vi "Get Download Progress.vi"(7 "Download Timeout (S)":u32, 8 "Error In":errorcluster, 11 "Download":T1) -> (0 "Error Out":errorcluster, 1 "Complete?":bool, 2 "Percent Complete":i32, 3 "Download":T1, 4 "Timeout?":bool)   [LabVIEW 2011, in "LVH-Toolbox.lvlib" / "LVH-Common.lvlib"]
doc: "Get progress of current download. If the download fails to progress during the timeout duration the download will be aborted.\n\nCall this VI in a loop after starting a download to monitor the download progress."
uses:
  LVH-Common.lvlib
  Private/Web/Type Defs/Download Task.ctl
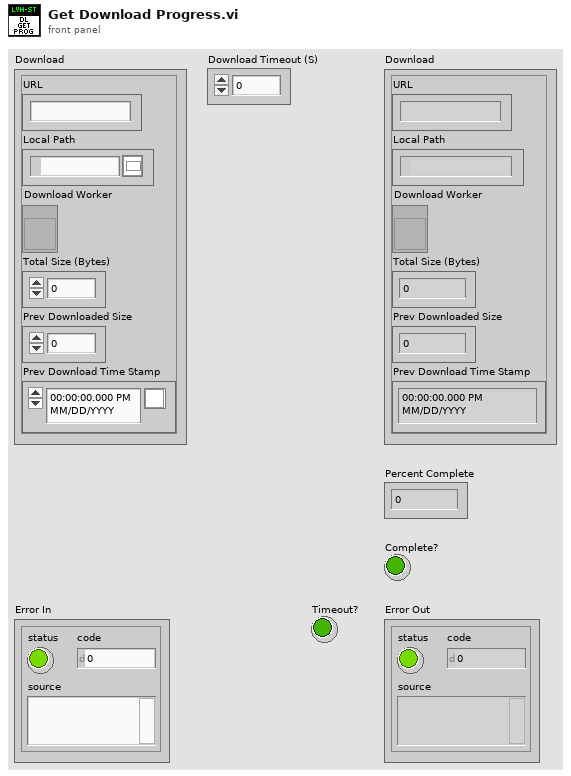
[diagram p1: front panel]
types:
  T1 = typedef "LVH-Toolbox.lvlib/LVH-Common.lvlib/Download Task.ctl" = cluster{"URL":string, "Local Path":path, "Download Worker":refnum<vi>, "Total Size (Bytes)":u64, "Prev Downloaded Size":u64, "Prev Download Time Stamp":timestamp}
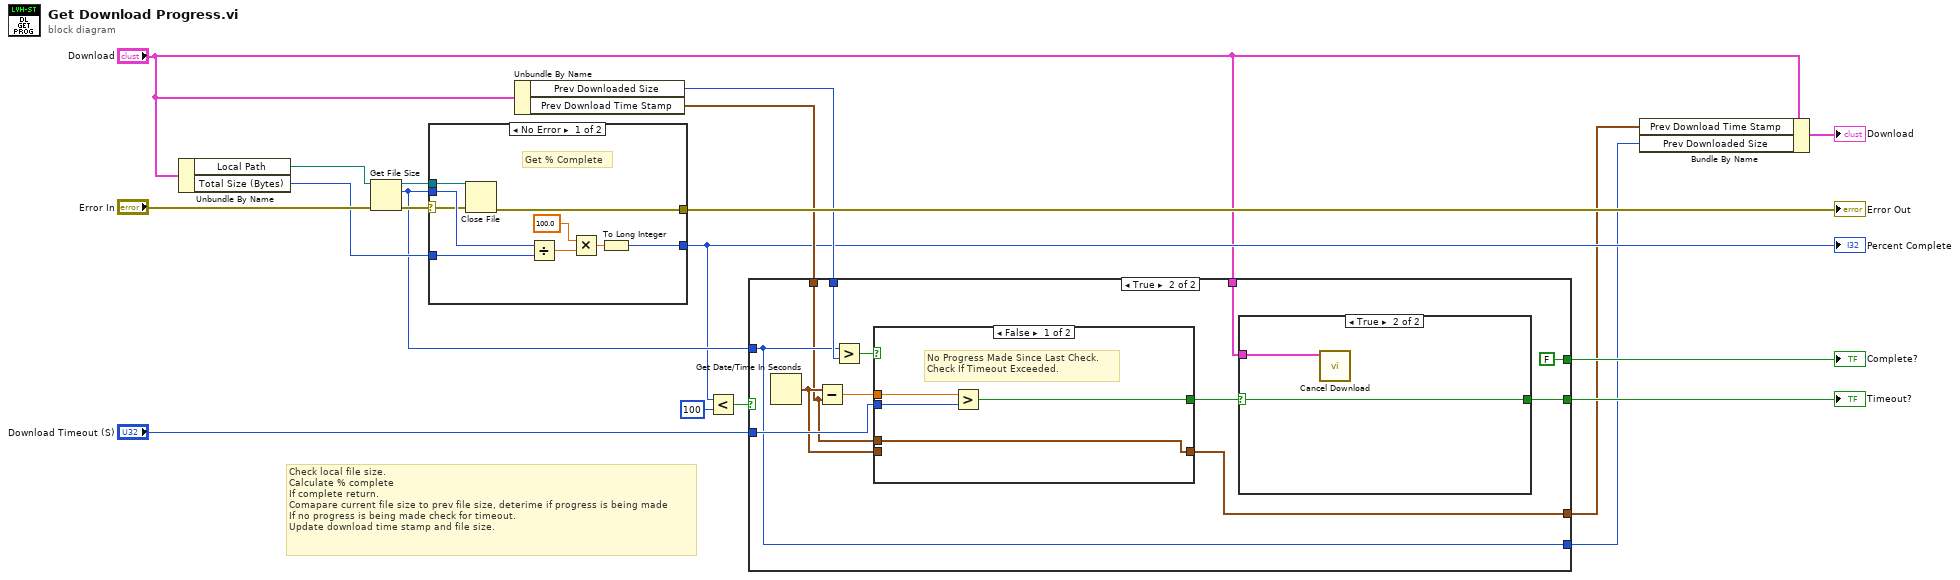
[diagram p0: block diagram]
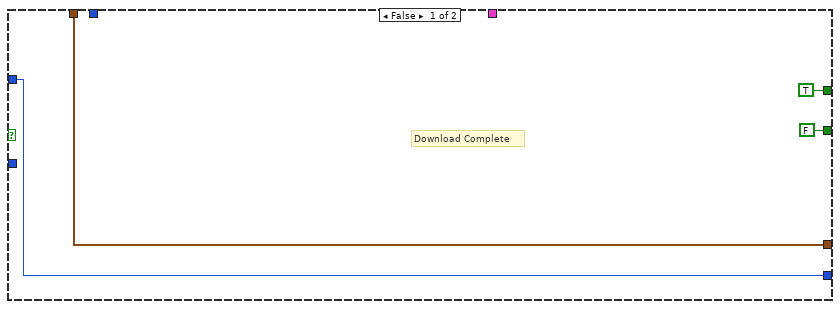
[diagram p2: hidden frame]
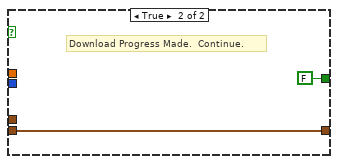
[diagram p4: hidden frame]
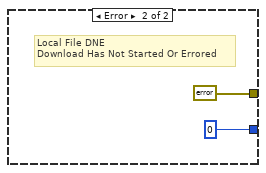
[diagram p5: hidden frame]
diagram:
  # "Check local file size.\nCalculate % complete\nIf complete return.\nComapare current file size to prev file size, deterime if progress is being made\nIf no progress is being made check for timeout.\nUpdate download time stamp and file size."
  n1 = Unbundle By Name("Download") -> ("Local Path"=w16:path, "Total Size (Bytes)"=w15:u64)
  n2 = Get File Size(file=w16, error in="Error In") -> (refnum out=w5:refnum<file>, size (in bytes)=w14:i64, 0:w17:errorcluster)
  n3 = case shown="No Error" w17 {
    selector: w17 -> [w21 _]
    tunnel: w14 -> [w28 _]
    tunnel: w5 -> [w24 _]
    tunnel: [w23 0] -> w8
    tunnel: [w22 errorcluster {"status"=FALSE, "code"=0, "source"=""} ("error out")] -> w18
    tunnel: w15 -> [w20 _]
    frame No Error {
      # "Get % Complete"
      n4 = Close File(refnum=w24, error in=w21) -> (error out=w22:errorcluster)  [unwired: 1 out]
      n5 = Divide(x=w28, y=w20) -> (x/y=w27:dbl)
      n6 = Multiply(x=100.0, y=w27) -> (x*y=w25:dbl)
      n7 = To Long Integer(number=w25) -> (32bit integer=w23:i32)
    }
    frame Error {
      # "Local File DNE\nDownload Has Not Started Or Errored"
    }
  }
  "Error Out" <- w18
  "Percent Complete" <- w8
  n8 = Unbundle By Name("Download") -> ("Prev Downloaded Size"=w11:u64, "Prev Download Time Stamp"=w10:timestamp)
  n9 = Less?(x=w8, y=100) -> (x < y?=w9:bool)
  n10 = case shown="True" w9 {
    tunnel: w14 -> [w32 w38]
    tunnel: "Download Timeout (S)" -> [_ w44]
    tunnel: [FALSE w42] -> w12
    tunnel: "Download" -> [_ w41]
    tunnel: w11 -> [_ w40]
    tunnel: w10 -> [w31 w35]
    tunnel: [TRUE FALSE] -> w6
    tunnel: [w31 w37] -> w2
    tunnel: [w32 w38] -> w1
    frame False {
      # "Download Complete"
    }
    frame True {
      n11 = Get Date/Time In Seconds() -> (seconds since 1Jan1904=w36:timestamp)
      n12 = Subtract(x=w36, y=w35) -> (x-y=w45:dbl)
      n13 = Greater?(x=w38, y=w40) -> (0:w46:bool)
      n14 = case shown="False" w46 {
        tunnel: w45 -> [w53 _]
        tunnel: w44 -> [w52 _]
        tunnel: [w51 FALSE] -> w43
        tunnel: [w50 w54] -> w37
        tunnel: w36 -> [_ w54]
        tunnel: w35 -> [w50 _]
        frame False {
          # "No Progress Made Since Last Check.\nCheck If Timeout Exceeded."
          n15 = Greater?(x=w53, y=w52) -> (0:w51:bool)
        }
        frame True {
          # "Download Progress Made.  Continue."
        }
      }
      n16 = case shown="True" w43 {
        selector: w43 -> [w47 w49]
        tunnel: [w47 w49] -> w42
        tunnel: w41 -> [_ w48]
        frame False {
          # "Download In Progress.  Continue"
        }
        frame True {
          n17 = call "Cancel Download.vi"("Download"=w48) -> ()  [unwired: 9 in, 2 out]
        }
      }
    }
  }
  "Timeout?" <- w12
  "Complete?" <- w6
  n18 = Bundle By Name(cluster="Download", "Prev Download Time Stamp"=w2, "Prev Downloaded Size"=w1) -> (→"Download":T1)
